vi "Example Add Numbers.vi"(8 "error in (no error)":errorcluster, 10 "y":dbl, 11 "x":dbl) -> (0 "error out":errorcluster)   [LabVIEW 2014]
uses:
  <vilib>/addons/_JKI Toolkits/Caraya/classes/Test/Test.lvclass
  <vilib>/addons/_JKI Toolkits/Caraya/classes/Assert/Assert.lvclass
panel:
  out "x+y":dbl
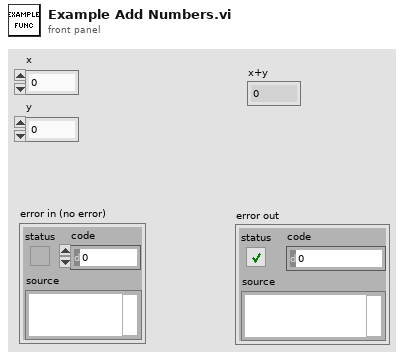
[diagram p1: front panel]
types:
  T1 = enum32{"Bad", "Idle", "Run top level", "Running"}
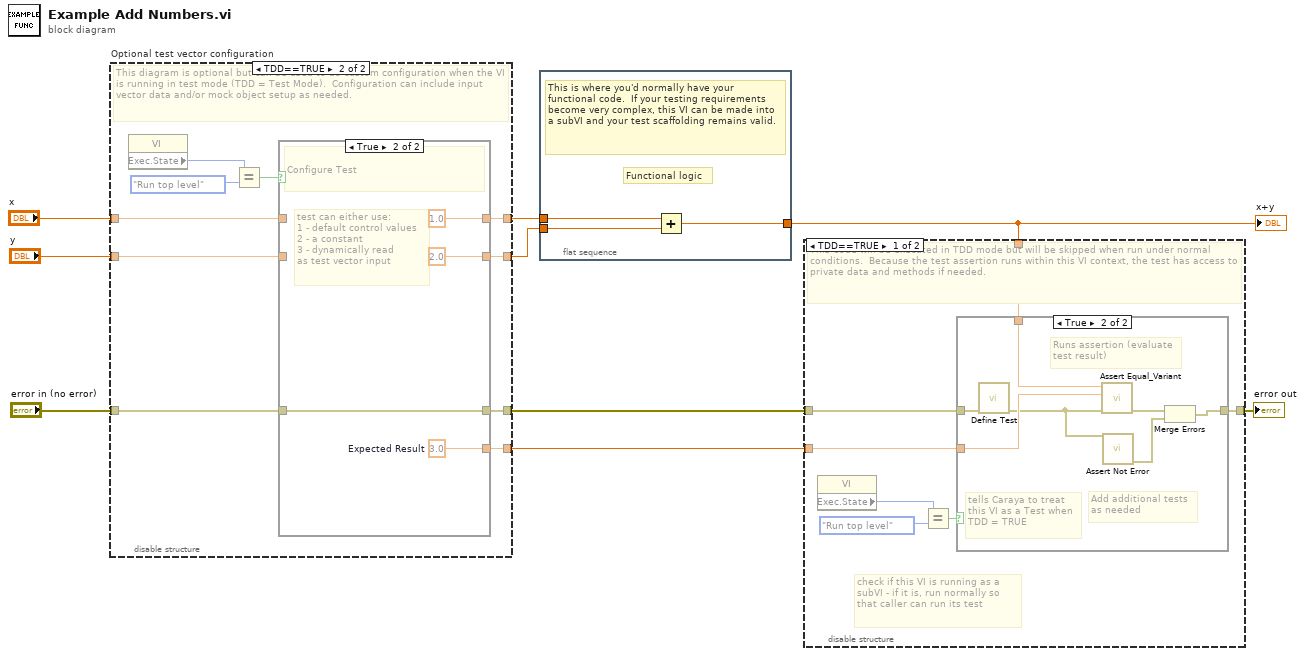
[diagram p0: block diagram]
diagram:
  n1 = disable-structure "Optional test vector configuration" shown="TDD==TRUE" {
    disable-tunnel: [w12 w22] -> w5
    disable-tunnel: "x" -> [w12 w17]
    disable-tunnel: [w11 w15] -> w3
    disable-tunnel: "error in (no error)" -> [w11 w14]
    disable-tunnel: "y" -> [w10 w16]
    disable-tunnel: [w10 w21] -> w4
    disable-tunnel: [_ w20] -> w1
    frame condition #0 (active) {
      # "Normal execution case use inputs passed into conn pane terminals"
    }
    frame condition #1 {
      # "This diagram is optional but can be used to do custom configuration when the VI is running in test mode (TDD = Test Mode).  Configuration can include input vector data and/or mock object setup as needed."
      n2 = property class="VI"() -> ("Exec.State"=w18:T1)  [unwired: 2 in, 2 out]
      n3 = Equal?(x=w18, y=T1."Run top level" ("Execution:State")) -> (x = y?=w13:bool)
      n4 = case shown="True" w13 {
        tunnel: [w25 1.0 ("x")] -> w22
        tunnel: [w24 2.0 ("y")] -> w21
        tunnel: [_ w27] -> w20
        tunnel: w17 -> [w25 _]
        tunnel: w16 -> [w24 _]
        tunnel: [w23 w26] -> w15
        tunnel: w14 -> [w23 w26]
        frame False {
          # "Another test is running this VI as a subVI so run normally"
        }
        frame True {
          w27 = 3.0  # Expected Result
          # "test can either use:\n1 - default control values\n2 - a constant\n3 - dynamically read \nas test vector input"
          # "Configure Test"
        }
      }
    }
  }
  n5 = flat-sequence {
    tunnel: w5 -> [w32]
    tunnel: w4 -> [w31]
    tunnel: [w30] -> w2
    frame #0 {
      # "Functional logic"
      # "This is where you'd normally have your functional code.  If your testing requirements become very complex, this VI can be made into a subVI and your test scaffolding remains valid."
      n6 = Add(x=w32, y=w31) -> (x+y=w30:dbl)
    }
  }
  n7 = disable-structure shown="TDD==TRUE" {
    disable-tunnel: w3 -> [w36 w48]
    disable-tunnel: [w39 w48] -> w9
    disable-tunnel: w2 -> [w38 _]
    disable-tunnel: w1 -> [w37 _]
    frame condition #0 {
      # "check if this VI is running as a subVI - if it is, run normally so that caller can run its test"
      # "This Code will be executed in TDD mode but will be skipped when run under normal conditions.  Because the test assertion runs within this VI context, the test has access to private data and methods if needed."
      n8 = property class="VI"() -> ("Exec.State"=w35:T1)  [unwired: 2 in, 2 out]
      n9 = Equal?(x=w35, y=T1."Run top level" ("Execution:State")) -> (x = y?=w33:bool)
      n10 = case shown="True" w33 {
        tunnel: [w40 w42] -> w39
        tunnel: w38 -> [_ w47]
        tunnel: w37 -> [_ w46]
        tunnel: w36 -> [w40 w45]
        frame False {
        }
        frame True {
          # "Add additional tests\nas needed"
          # "Runs assertion (evaluate\ntest result)"
          # "tells Caraya to treat\nthis VI as a Test when\nTDD = TRUE"
          n11 = call <vilib>:"Define Test.vi"("error in (no error)"=w45) -> ("error out"=w43:errorcluster)  [unwired: 10 in]
          n12 = call <vilib>:"Assert Equal_Variant.vi"("error in (no error)"=w43, "Y"=w46, "X"=w47) -> ("error out"=w44:errorcluster)  [unwired: 8 in]
          n13 = call <vilib>:"Assert Not Error.vi"("Not Error?"=w43) -> ("error out"=w41:errorcluster)  [unwired: 10 in]
          n14 = Merge Errors(w44, w41) -> (w42:errorcluster)
        }
      }
    }
    frame condition #1 (active) {
      # "When not running a test (or when built into EXE) this code is stripped out by LabVIEW compiler so there is no performance penalty or dependency on Caraya in the built application."
    }
  }
  "error out" <- w9
  "x+y" <- w2
